vi "globe vari.vi"() -> ()   [LabVIEW 2023]
panel:
  in  "路径":path
  in  "CP2保温2":dbl
  in  "CP2保温1":dbl
  in  "Q保温":dbl
  in  "CP1保温 2":dbl
  in  "CP1保温1":dbl
  in  "恒温槽温度":dbl
  in  "天平控制串口":refnum<visa-resource-name>
  in  "蠕动泵控制串口":refnum<visa-resource-name>
  in  "搅拌桨控制串口":refnum<visa-resource-name>
  out "电源控制串口":refnum<visa-resource-name>
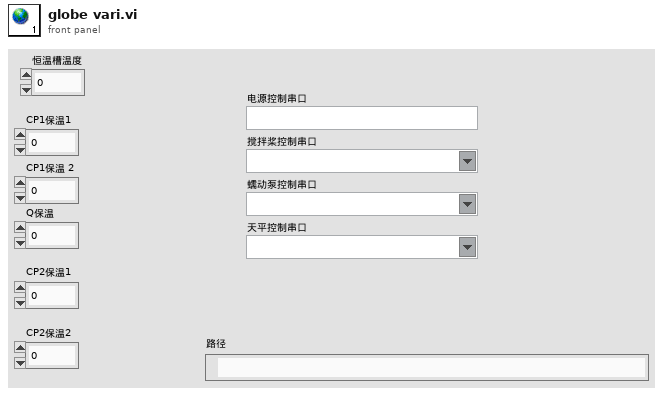
[diagram p1: front panel]
diagram:
